vi "Set Timekeeper Card.vi"(8 "error in (no error)":errorcluster, 11 "RT Data Cluster in":T1={"Timekeeper hdl"="", "clkDisc session"=variant, "Compiled Data"={"SyncMod?"=FALSE, "SyncMod"="", "ConnectionSettings"={"Mode"=enum."Generate sample clock", "pxitrig"=FALSE, "pfi0"=FALSE, "pfi1"=FALSE, "pfi2"=FALSE, "External Pin"=enum."PFI0", "Routes"=[]}, "TimeKeeper"="", "ScanOffset(%)"=0.0, "StartDelay(s)"=0, "Time Ref Settings"={"Time Reference"=enum."GPS", "Priority 1"=0, "Priority 2"=0, "IRIG type"=enum."IRIGB AM", "Terminal"="", "PPSSetTime"=FALSE, "Start Time"=timestamp(0 s since 1904-01-01)}, "FIFO Locations"={"BoardTime"=[], "Status"=[]}}, "OutputsData"=[], "OutputsFIFO"=refnum, "Scan Period"=0, "Timekeeper type"=enum."6683", "SyncMod type"=enum."6683", "SyncMod hdl"=""} {"Compiled Data"."Time Ref Settings"."Priority 2" min=0 max=255; "Compiled Data"."Time Ref Settings"."Priority 1" min=0 max=255}) -> (0 "error out":errorcluster, 3 "RT Data Cluster out":T1={"Timekeeper hdl"="", "clkDisc session"=variant, "Compiled Data"={"SyncMod?"=FALSE, "SyncMod"="", "ConnectionSettings"={"Mode"=enum."Generate sample clock", "pxitrig"=FALSE, "pfi0"=FALSE, "pfi1"=FALSE, "pfi2"=FALSE, "External Pin"=enum."PFI0", "Routes"=[]}, "TimeKeeper"="", "ScanOffset(%)"=0.0, "StartDelay(s)"=0, "Time Ref Settings"={"Time Reference"=enum."GPS", "Priority 1"=0, "Priority 2"=0, "IRIG type"=enum."IRIGB AM", "Terminal"="", "PPSSetTime"=FALSE, "Start Time"=timestamp(0 s since 1904-01-01)}, "FIFO Locations"={"BoardTime"=[], "Status"=[]}}, "OutputsData"=[], "OutputsFIFO"=refnum, "Scan Period"=0, "Timekeeper type"=enum."6683", "SyncMod type"=enum."6683", "SyncMod hdl"=""} {"Compiled Data"."Time Ref Settings"."Priority 2" min=0 max=255; "Compiled Data"."Time Ref Settings"."Priority 1" min=0 max=255})   [LabVIEW 2015, in "NI Synchronization Engine.lvlib"]
uses:
  NI Synchronization Engine.lvlib
  RT Data Cluster.ctl
  mdevClkDisc.llb/_clkDisc_session.ctl
  Shared/Compiled Data.ctl
  Shared/Connection Settings.ctl
  Shared/Mode.ctl
  Shared/External Pin.ctl
  Shared/Routes.ctl
  Shared/Route.ctl
  Shared/Time Ref Settings.ctl
  Shared/Time Reference.ctl
  Shared/IRIG Type.ctl
  timekeeper type.ctl
  <vilib>/Utility/config.llb/NI_LVConfig.lvlib
  <vilib>/Utility/config.llb/Read Key (String).vi
  <vilib>/Utility/config.llb/Write Key (String).vi
  Shared/NI Synchronization Shared.lvlib
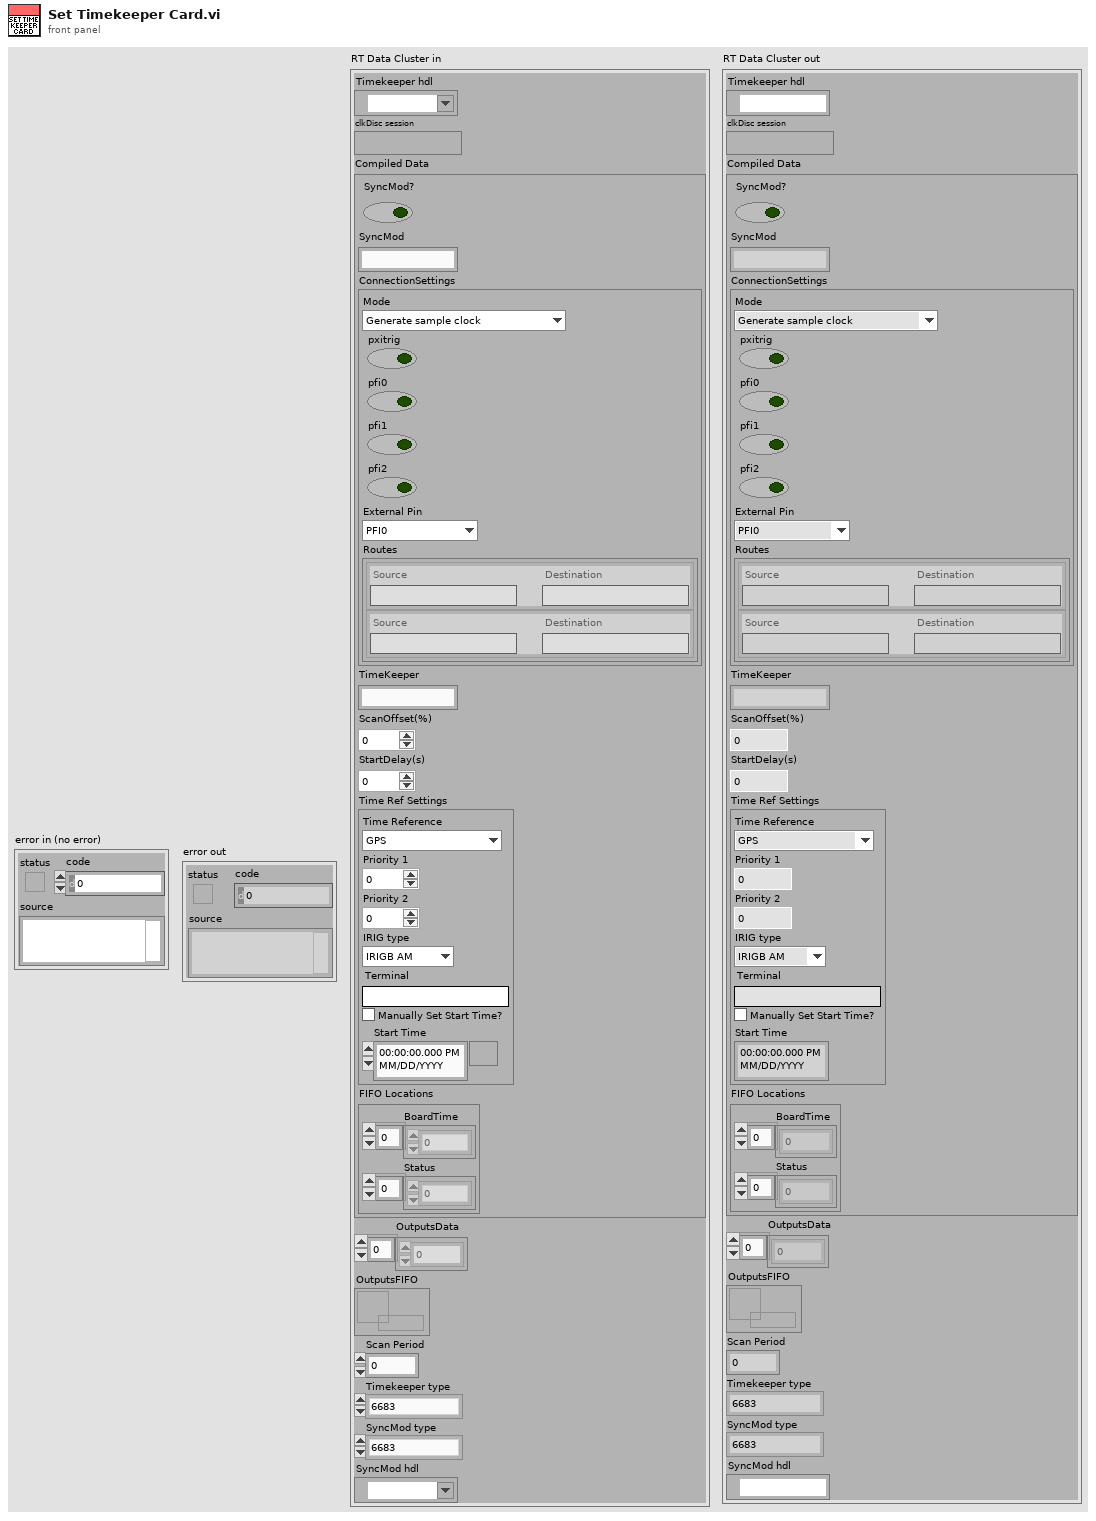
[diagram p1: front panel]
types:
  T1 = typedef "NI Synchronization Engine.lvlib/RT Data Cluster.ctl" = cluster{"Timekeeper hdl":refnum<k15>, "clkDisc session":T2, "Compiled Data":T3, "OutputsData":dbl[], "OutputsFIFO":refnum<k33>, "Scan Period":u32, "Timekeeper type":T12, "SyncMod type":T12, "SyncMod hdl":refnum<k15>}
  T2 = typedef "_clkDisc_session.ctl" = variant
  T3 = typedef "NI Synchronization Shared.lvlib/Compiled Data.ctl" = cluster{"SyncMod?":bool, "SyncMod":string, "ConnectionSettings":T4, "TimeKeeper":string, "ScanOffset(%)":dbl, "StartDelay(s)":u16, "Time Ref Settings":T9, "FIFO Locations":cluster{"BoardTime":i32[], "Status":i32[]}}
  T4 = typedef "NI Synchronization Shared.lvlib/Connection Settings.ctl" = cluster{"Mode":T5, "pxitrig":bool, "pfi0":bool, "pfi1":bool, "pfi2":bool, "External Pin":T6, "Routes":T7}
  T5 = typedef "NI Synchronization Shared.lvlib/Mode.ctl" = enum16{"Generate sample clock", "Route sample clock out of chassis", "Route sample clock into chassis", "Custom routes"}
  T6 = typedef "NI Synchronization Shared.lvlib/External Pin.ctl" = enum16{"PFI0", "PFI1", "PFI2"}
  T7 = typedef "NI Synchronization Shared.lvlib/Routes.ctl" = T8[]
  T8 = typedef "NI Synchronization Shared.lvlib/Route.ctl" = cluster{"Source":string, "Destination":string}
  T9 = typedef "NI Synchronization Shared.lvlib/Time Ref Settings.ctl" = cluster{"Time Reference":T10, "Priority 1":i32, "Priority 2":i32, "IRIG type":T11, "Terminal":string, "PPSSetTime":bool, "Start Time":timestamp}
  T10 = typedef "NI Synchronization Shared.lvlib/Time Reference.ctl" = enum16{"GPS", "IRIG", "PPS", "1588 Ordinary Clock", "802.1AS", "PXI Chassis Clock", "Free Running (Internal)"}
  T11 = typedef "NI Synchronization Shared.lvlib/IRIG Type.ctl" = enum16{"IRIGB DC", "IRIGB AM"}
  T12 = typedef "NI Synchronization Engine.lvlib/timekeeper type.ctl" = enum16{"6683", "6683H", "6682", "6682H", "non-timekeeper", "timekeeper"}
  T13 = typedef "NI_LVConfig.lvlib/Config Data RefNum.ctl" = refnum<k1>
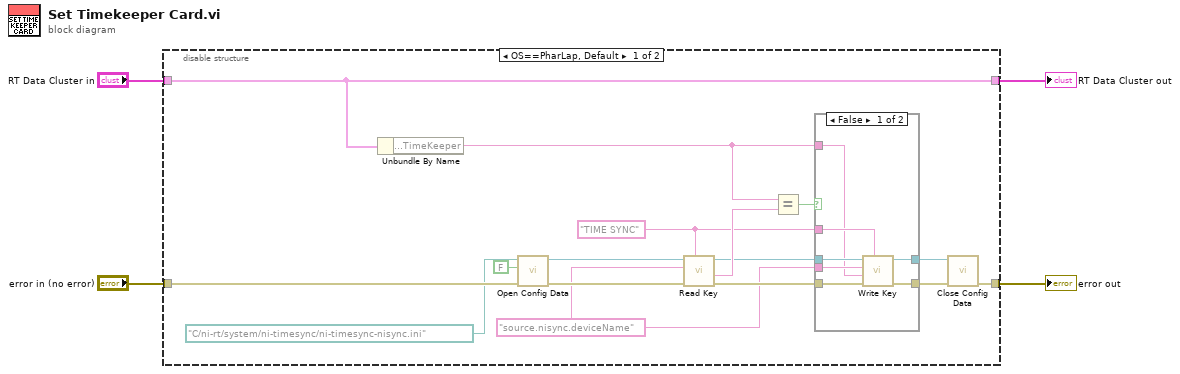
[diagram p0: block diagram]
diagram:
  n1 = disable-structure shown="OS==PharLap, Default" {
    disable-tunnel: "error in (no error)" -> [w20 w30]
    disable-tunnel: "RT Data Cluster in" -> [w5 w31]
    disable-tunnel: [w6 w30] -> w2
    disable-tunnel: [w5 w31] -> w1
    frame condition #0 {
      w10 = "source.nisync.deviceName" ("section")
      w11 = "TIME SYNC" ("section")
      n2 = Unbundle By Name(w5) -> ("Compiled Data.TimeKeeper"=w9:string)
      n3 = call <vilib>:"Open Config Data.vi"("error in (no error)"=w20, "create file if necessary (T)"=FALSE, "configuration file path"=path "C:/ni-rt/system/ni-timesync/ni-timesync-nisync.ini") -> ("error out"=w17:errorcluster, "refnum"=w16:T13)  [unwired: 6 in, 1 out]
      n4 = call-poly <vilib>:"Read Key.vi"("section"=w11, "error in (no error)"=w17, "key"=w10, "refnum"=w16) -> ("error out"=w15:errorcluster, "value"=w14:string, "refnum out"=w12:T13)  [unwired: 4 in, 1 out]
      n5 = Equal?(x=w9, y=w14) -> (x = y?=w13:bool)
      n6 = case shown="False" w13 {
        tunnel: w15 -> [w27 w28]
        tunnel: w12 -> [w26 w29]
        tunnel: w11 -> [w25 _]
        tunnel: w10 -> [w24 _]
        tunnel: w9 -> [w23 _]
        tunnel: [w22 w28] -> w8
        tunnel: [w21 w29] -> w7
        frame False {
          n7 = call-poly <vilib>:"Write Key.vi"("section"=w25, "error in (no error)"=w27, "value"=w23, "key"=w24, "refnum"=w26) -> ("error out"=w22:errorcluster, "refnum out"=w21:T13)  [unwired: 4 in, 1 out]
        }
        frame True {
        }
      }
      n8 = call <vilib>:"Close Config Data.vi"("error in (no error)"=w8, "refnum"=w7) -> ("error out"=w6:errorcluster)  [unwired: 8 in, 1 out]
    }
    frame condition #1 (active) {
      # "Current behavior is to use the timing card in the lowest slot number"
    }
  }
  "error out" <- w2
  "RT Data Cluster out" <- w1
